vi "Check TTL-Only Status.vi"(0 "State in":refnum<class "State.lvclass">, 5 "Num linking to this state":i32, 7 "Action":T1, 9 "Start state":bool, 11 "error in (no error)":errorcluster) -> (4 "State out":refnum<class "State.lvclass">, 6 "accepted":bool, 10 "TTL-only changed":bool, 15 "error out":errorcluster)   [LabVIEW 2015, in "State.lvclass"]
uses:
  State.lvclass
  Typedefs/Tosca-Termination Condition Action.ctl
  State.lvclass/State.ctl
  Timeout/Timeout.lvclass/Timeout.ctl
  Timeout/Read Link to.vi
  Timeout/Timeout.lvclass
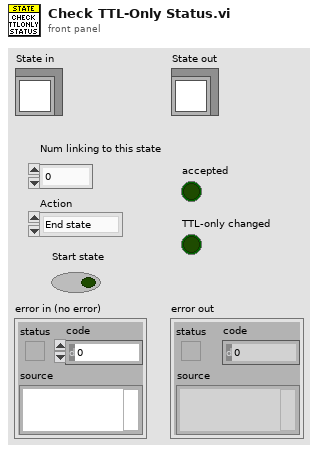
[diagram p1: front panel]
types:
  T1 = typedef "Tosca-Termination Condition Action.ctl" = enum16{"End state", "Complete state", "TTL only"}
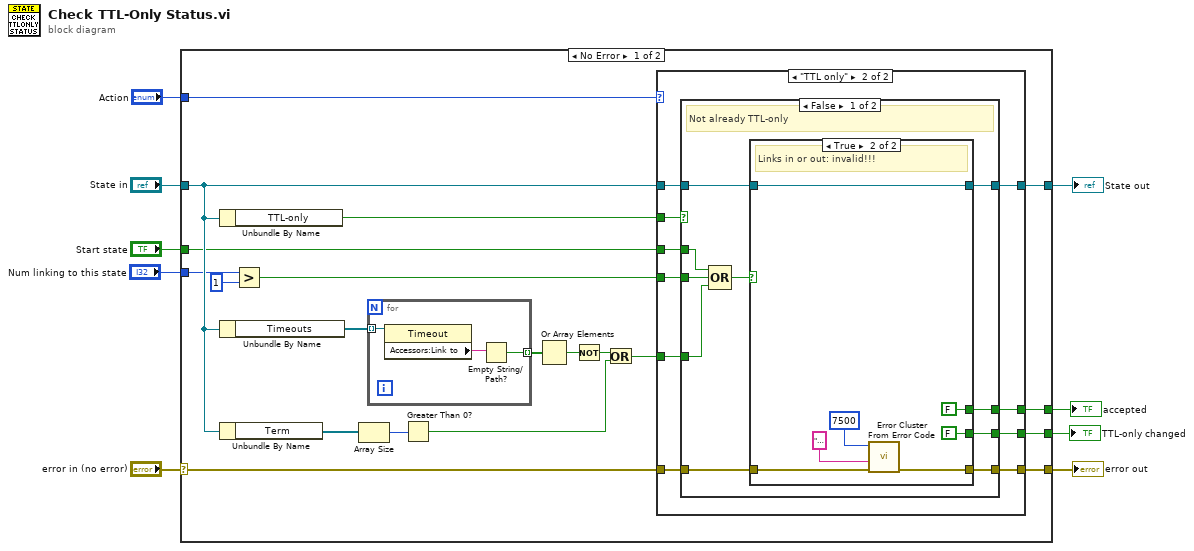
[diagram p0: block diagram]
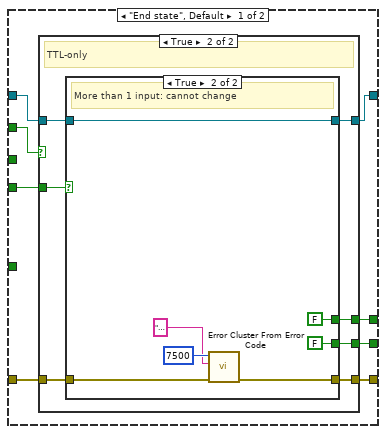
[diagram p2: hidden frame]
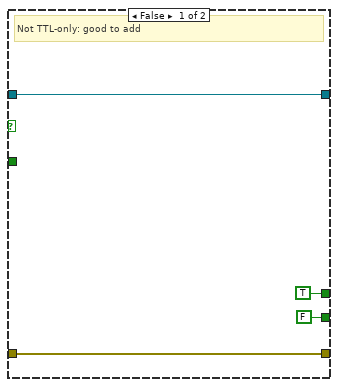
[diagram p3: hidden frame]
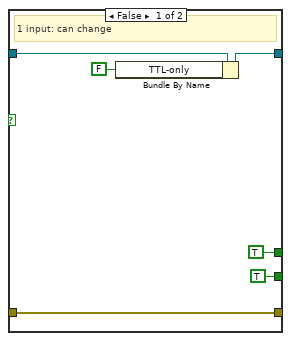
[diagram p4: hidden frame]
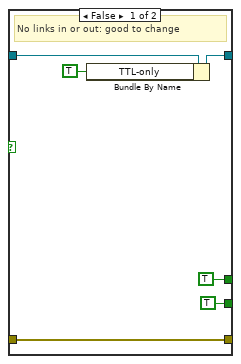
[diagram p5: hidden frame]
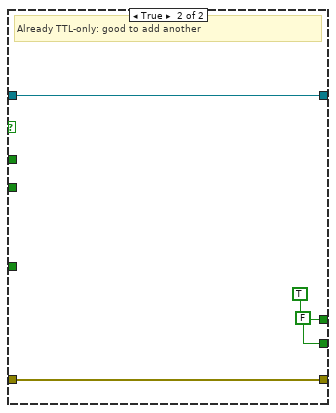
[diagram p6: hidden frame]
diagram:
  n1 = case shown="No Error" "error in (no error)" {
    selector: "error in (no error)" -> [w11 w103]
    tunnel: [w12 w103] -> w8
    tunnel: [w20 w102] -> w6
    tunnel: "State in" -> [w19 w102]
    tunnel: "Action" -> [w22 _]
    tunnel: "Num linking to this state" -> [w17 _]
    tunnel: [w14 _] -> w3
    tunnel: [w13 _] -> w2
    tunnel: "Start state" -> [w10 _]
    frame No Error {
      n2 = Unbundle By Name(w19) -> ("TTL-only"=w21:bool)
      n3 = Unbundle By Name(w19) -> ("Timeouts"=w29:refnum<class "Timeout.lvclass">[])
      n4 = Unbundle By Name(w19) -> ("Term"=w28:refnum<class "Termination.lvclass">[])
      n5 = Greater?(x=w17, y=1) -> (0:w16:bool)
      n6 = Array Size(array=w28) -> (size(s)=w25:i32)
      n7 = for {
        tunnel: w29 -> [w101] mode=indexing
        tunnel: [w99] -> w27 mode=indexing
        n8 = property class="Timeout"(reference=w101) -> ("Accessors:Link to"=w100:string)  [unwired: 1 in, 2 out]
        n9 = Empty String/Path?(string/path=w100) -> (empty?=w99:bool)
      }
      n10 = Greater Than 0?(x=w25) -> (x > 0?=w23:bool)
      n11 = Or Array Elements(Boolean array=w27) -> (logical OR=w26:bool)
      n12 = Not(x=w26) -> (.not. x?=w24:bool)
      n13 = Or(x=w24, y=w23) -> (x .or. y?=w18:bool)
      n14 = case shown="\"TTL only\"" w22 {
        tunnel: w21 -> [w35 w71]
        tunnel: [w37 w70] -> w20
        tunnel: w19 -> [w36 w69]
        tunnel: w18 -> [_ w67]
        tunnel: w16 -> [w32 w68]
        tunnel: [w34 w66] -> w14
        tunnel: [w33 w65] -> w13
        tunnel: [w31 w64] -> w12
        tunnel: w11 -> [w30 w63]
        tunnel: w10 -> [_ w62]
        frame "End state", Default {
          n15 = case shown="True" w35 {
            tunnel: [w41 w48] -> w37
            tunnel: w36 -> [w41 w47]
            tunnel: [TRUE w45] -> w34
            tunnel: [FALSE w44] -> w33
            tunnel: w32 -> [_ w46]
            tunnel: [w38 w42] -> w31
            tunnel: w30 -> [w38 w43]
            frame False {
              # "Not TTL-only: good to add"
            }
            frame True {
              # "TTL-only"
              n16 = case shown="True" w46 {
                tunnel: [w53 w61] -> w48
                tunnel: w47 -> [w54 w61]
                tunnel: [TRUE FALSE] -> w45
                tunnel: [TRUE FALSE] -> w44
                tunnel: w43 -> [w49 w57]
                tunnel: [w49 w56] -> w42
                frame False {
                  # "1 input: can change"
                  n17 = Bundle By Name(cluster=w54, "TTL-only"=FALSE ("Serialized.TTL-only")) -> (w53:refnum<class "State.lvclass">)
                }
                frame True {
                  # "More than 1 input: cannot change"
                  n18 = call <vilib>:"Error Cluster From Error Code.vi"("error in (no error)"=w57, "error message (\"\")"="The state linked to must remain \"TTL-only\" because\n->it has another input that is set to TTL-only" ("error message (\"\")"), "error code (0)"=7500) -> ("error out"=w56:errorcluster)  [unwired: 6 in]
                }
              }
            }
          }
        }
        frame "TTL only" {
          n19 = case shown="False" w71 {
            tunnel: [w77 w98] -> w70
            tunnel: w69 -> [w78 w98]
            tunnel: w68 -> [w81 _]
            tunnel: w67 -> [w80 _]
            tunnel: [w76 TRUE] -> w66
            tunnel: [w75 FALSE] -> w65
            tunnel: [w74 w95] -> w64
            tunnel: w63 -> [w73 w95]
            tunnel: w62 -> [w72 _]
            frame False {
              # "Not already TTL-only"
              n20 = Compound Arithmetic op=OR(w72, w81, w80) -> (w79:bool)
              n21 = case shown="True" w79 {
                tunnel: w78 -> [w87 w94]
                tunnel: [w84 w94] -> w77
                tunnel: [TRUE FALSE] -> w76
                tunnel: [TRUE FALSE] -> w75
                tunnel: [w82 w90] -> w74
                tunnel: w73 -> [w82 w91]
                frame False {
                  # "No links in or out: good to change"
                  n22 = Bundle By Name(cluster=w87, "TTL-only"=TRUE ("Serialized.TTL-only")) -> (w84:refnum<class "State.lvclass">)
                }
                frame True {
                  # "Links in or out: invalid!!!"
                  n23 = call <vilib>:"Error Cluster From Error Code.vi"("error in (no error)"=w91, "error message (\"\")"="The state linked to cannot be \"TTL-only\" because \n->it links to other states, or \n->it already has inputs that are not TTL-only, or\n->it is the start state\n" ("error message (\"\")"), "error code (0)"=7500) -> ("error out"=w90:errorcluster)  [unwired: 6 in]
                }
              }
            }
            frame True {
              # "Already TTL-only: good to add another"
            }
          }
        }
      }
    }
    frame Error {
    }
  }
  "error out" <- w8
  "State out" <- w6
  "TTL-only changed" <- w2
  "accepted" <- w3
